vi "Make Section Images.vi"(8 "Error In":errorcluster, 9 "Footer Info":T1, 10 "Main Body Info":T1, 11 "Header Info":T1) -> (0 "Error Out":errorcluster, 1 "Footer Image":T2, 2 "Main Body Image":T2, 3 "Header Image":T2)   [LabVIEW 2018, in "Image Management.lvlib"]
uses:
  Image Management.lvlib
  <vilib>/vision/Image Controls.llb/IMAQ Image.ctl
  receipt parsing/Section Info--cluster.ctl
  Action.ctl
  receipt parsing/Receipt Parsing.lvlib
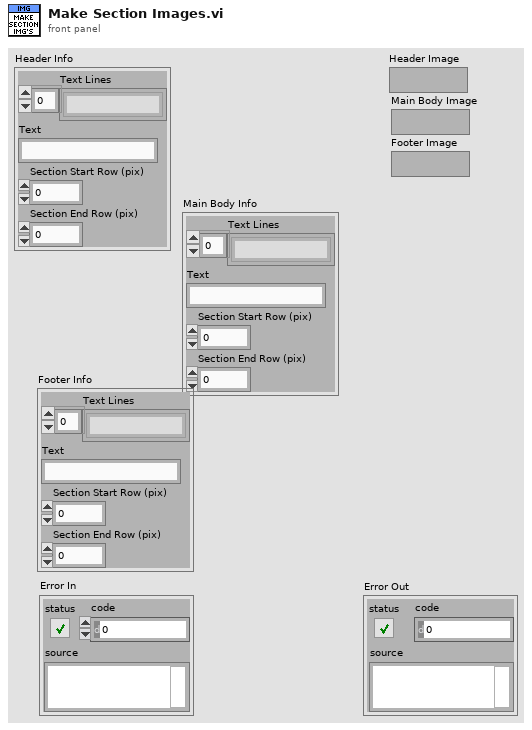
[diagram p1: front panel]
types:
  T1 = typedef "Receipt Parsing.lvlib/Section Info--cluster.ctl" = cluster{"Text Lines":string[], "Text":string, "Section Start Row (pix)":i32, "Section End Row (pix)":i32}
  T2 = typedef "IMAQ Image.ctl" = refnum<image>
  T3 = cluster{"Header Image":T2, "Main Body Image":T2, "Footer Image":T2}
  T4 = typedef "Image Management.lvlib/Action.ctl" = enum16{"Init", "Output Image Path", "Open Image in Default Program", "Find Linespaces", "Get Image Size (pixels)", "Draw ROIs", "Make Section Images", "Close"}
  T5 = cluster{"Header Info":T1, "Main Body Info":T1, "Footer Info":T1}
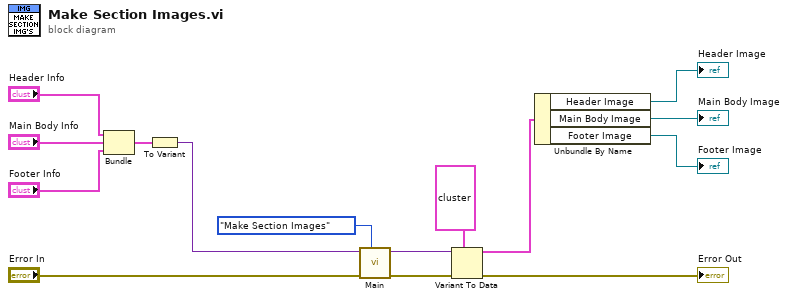
[diagram p0: block diagram]
diagram:
  n1 = Bundle("Header Info"="Header Info", "Main Body Info"="Main Body Info", "Footer Info"="Footer Info") -> (w5:T5)  [unwired: 1 in]
  n2 = To Variant(anything=w5) -> (Variant=w6:variant)
  n3 = call "Main.vi"("Action"=Action."Make Section Images", "Error In"="Error In", "Data in"=w6) -> ("Error Out"=w14:errorcluster, "Output"=w15:variant)  [unwired: 7 in]
  n4 = Variant To Data(error in=w14, type=T3 {"Header Image"=refnum, "Main Body Image"=refnum, "Footer Image"=refnum} ("cluster"), Variant=w15) -> (data=w10:T3, error out=→"Error Out":errorcluster)
  n5 = Unbundle By Name(w10) -> ("Header Image"=→"Header Image":T2, "Main Body Image"=→"Main Body Image":T2, "Footer Image"=→"Footer Image":T2)
